vi "lvstyx_read_all_path_float.vi"(7 "Log? (T)":bool=TRUE, 8 "error in (no error)":errorcluster, 10 "path":string, 11 "client ptr":u32) -> (0 "error out":errorcluster, 2 "double":dbl, 3 "dup client ptr":u32)   [LabVIEW 2010, in "lib1299.lvlib"]
uses:
  lib1299.lvlib
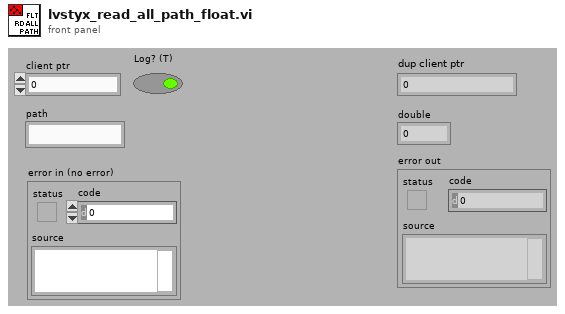
[diagram p1: front panel]
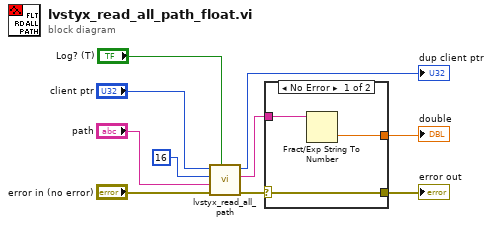
[diagram p0: block diagram]
diagram:
  n1 = call "lvstyx_read_all_path.vi"("Log? (T)"="Log? (T)", "error in (no error)"="error in (no error)", "path"="path", "lim"=16, "client ptr"="client ptr") -> ("error out"=w10:errorcluster, "buf"=w9:string, "dup client ptr"=→"dup client ptr":u32)  [unwired: 4 in]
  n2 = case shown="No Error" w10 {
    selector: w10 -> [w12 w14]
    tunnel: w9 -> [w13 _]
    tunnel: [w12 w14] -> w6
    tunnel: [w11 _] -> w2
    frame No Error {
      n3 = Fract/Exp String To Number(string=w13) -> (number=w11:dbl)  [unwired: 3 in, 1 out]
    }
    frame Error {
    }
  }
  "error out" <- w6
  "double" <- w2
